vi "Calc CIC Scaling Factor.vi"(11 "M":i32) -> (3 "shift":i32)   [LabVIEW 2018, in "Lock-In Amplifier Example Host.lvlib"]
uses:
  Lock-In Amplifier Example Host.lvlib
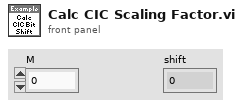
[diagram p1: front panel]
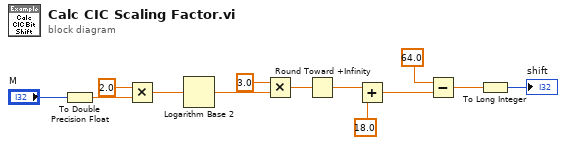
[diagram p0: block diagram]
diagram:
  n1 = To Double Precision Float(number="M") -> (double precision float=w2:dbl)
  n2 = Multiply(x=2.0, y=w2) -> (x*y=w11:dbl)
  n3 = Logarithm Base 2(1:w11) -> (0:w10:dbl)
  n4 = Multiply(x=3.0, y=w10) -> (x*y=w9:dbl)
  n5 = Round Toward +Infinity(x=w9) -> (ceil(x): smallest int >= x=w7:dbl)
  n6 = Add(x=w7, y=18.0) -> (x+y=w8:dbl)
  n7 = Subtract(x=64.0, y=w8) -> (x-y=w3:dbl)
  n8 = To Long Integer(number=w3) -> (32bit integer=→"shift":i32)
